vi "replace_position.vi"(2 "Position":cluster{"x":dbl, "y":dbl, "z":dbl}, 3 "Spot in":T1={"Position"={"x"=0.0, "y"=0.0, "z"=0.0}, "Intensity"=1.0, "Vortex Charge"=0, "Phase"=0.0, "NA Position"={"x"=0.0, "y"=0.0, "r"=1.0}, "Line Trapping"={"Vector"={"x"=0.0, "y"=0.0, "z"=0.0}, "Phase Gradient"=0.0}, "Amplitude Correction"=0.0} {"Amplitude Correction" step=0.1; "Line Trapping"."Phase Gradient" step=0.05; "Line Trapping"."Vector"."x" step=1e-06 format="%#_6p"; "Line Trapping"."Vector"."y" step=1e-06 format="%#_6p"; "Line Trapping"."Vector"."z" step=1e-06 format="%#_6p"; "NA Position"."r" step=1e-06; "NA Position"."y" step=1e-06; "NA Position"."x" step=1e-06; "Position"."z" step=1e-06; "Position"."y" step=1e-06; "Position"."x" step=1e-06; "Phase" step=0.7753; "Intensity" step=0.1}) -> (0 "Spot":T1={"Position"={"x"=0.0, "y"=0.0, "z"=0.0}, "Intensity"=0.0, "Vortex Charge"=0, "Phase"=0.0, "NA Position"={"x"=0.0, "y"=0.0, "r"=1.0}, "Line Trapping"={"Vector"={"x"=0.0, "y"=0.0, "z"=0.0}, "Phase Gradient"=0.0}, "Amplitude Correction"=0.0} {"Amplitude Correction" step=0.1; "Line Trapping"."Phase Gradient" step=0.05; "Line Trapping"."Vector"."x" step=1e-06 format="%#_6p"; "Line Trapping"."Vector"."y" step=1e-06 format="%#_6p"; "Line Trapping"."Vector"."z" step=1e-06 format="%#_6p"; "NA Position"."r" step=1e-06; "NA Position"."y" step=1e-06; "NA Position"."x" step=1e-06; "Position"."z" step=1e-06; "Position"."y" step=1e-06; "Position"."x" step=1e-06; "Phase" step=0.7753; "Intensity" step=0.1})   [LabVIEW 2010]
doc: "Replace the position in a spot."
uses:
  spot.ctl
  line_trapping.ctl
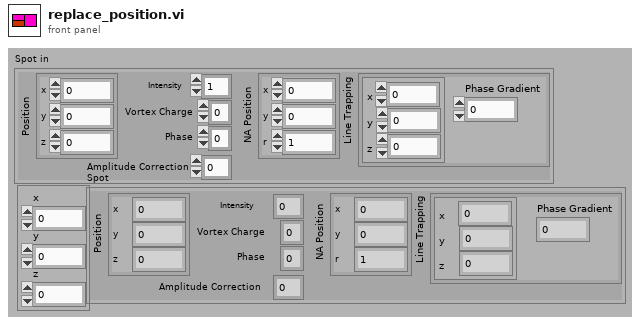
[diagram p1: front panel]
types:
  T1 = typedef "spot.ctl" = cluster{"Position":cluster{"x":dbl, "y":dbl, "z":dbl}, "Intensity":dbl, "Vortex Charge":i8, "Phase":dbl, "NA Position":cluster{"x":dbl, "y":dbl, "r":dbl}, "Line Trapping":T2, "Amplitude Correction":dbl}
  T2 = typedef "line_trapping.ctl" = cluster{"Vector":cluster{"x":dbl, "y":dbl, "z":dbl}, "Phase Gradient":dbl}
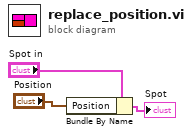
[diagram p0: block diagram]
diagram:
  n1 = Bundle By Name(cluster="Spot in", "Position"="Position") -> (→"Spot":T1)
